vi "Find Rows of Dragged Items.vi"(10 "Dragged Items":string[](array[string]), 11 "ListBox Strings":string[](array[string])) -> (3 "Rows":i32[](array[numeric]))   [LabVIEW 2011]
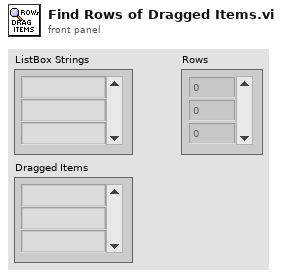
[diagram p1: front panel]
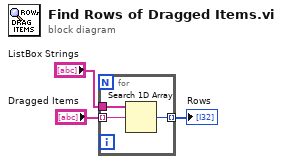
[diagram p0: block diagram]
diagram:
  n1 = for {
    tunnel: "Dragged Items" -> [w5] mode=indexing
    tunnel: "ListBox Strings" -> [w6]
    tunnel: [w4] -> w1 mode=indexing
    n2 = Search 1D Array(1D array=w6, element=w5) -> (index of element=w4:i32)  [unwired: 1 in]
  }
  "Rows" <- w1
